vi "StringToArray.vi"(11 "write buffer":string) -> (3 "Array":string[](array[string]))   [LabVIEW 2022 SP3]
uses:
  <vilib>/Utility/error.llb/Trim Whitespace One-Sided.vi
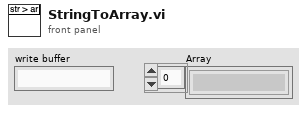
[diagram p1: front panel]
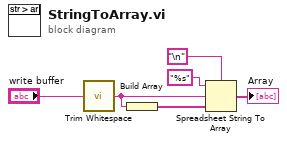
[diagram p0: block diagram]
diagram:
  n1 = call <vilib>:"Trim Whitespace.vi"("string"="write buffer") -> ("trimmed string"=w6:string)  [unwired: 1 in]
  n2 = Build Array(w6) -> (w1:string[])
  n3 = Spreadsheet String To Array(delimiter (Tab)="\n" ("regular expression"), format string="%s", spreadsheet string=w6, array type (2D Dbl)=w1) -> (array=→"Array":string[])
